vi "Construct.vi"(7 "ColumnMapping":string[][](array[string]), 8 "Error in (no error)":errorcluster, 9 "Table":string, 10 "Database":T1) -> (0 "Error out":errorcluster, 3 "LogWriterDb out":refnum<class "LogWriterDb.lvclass">)   [LabVIEW 2011, in "LogWriterDb.lvclass"]
uses:
  LogWriterDb.lvclass
  <vilib>/addons/database/Connection.llb/Conn ObjectReference.ctl
  LogWriterDb.lvclass/LogWriterDb.ctl
  <vilib>/addons/database/NI_Database_API.lvlib
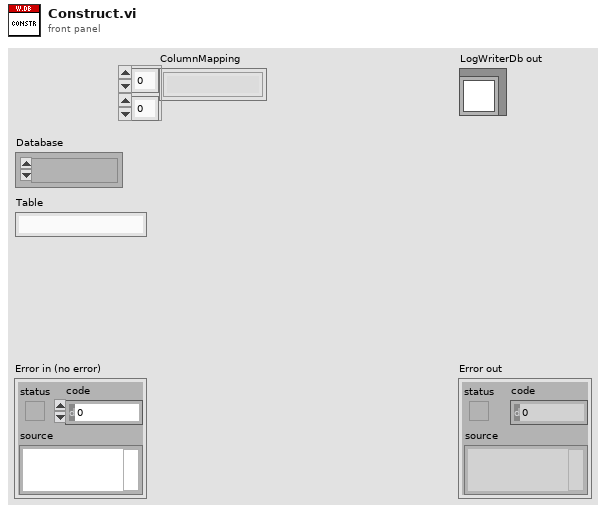
[diagram p1: front panel]
types:
  T1 = typedef "NI_Database_API.lvlib/Conn ObjectReference.ctl" = refnum<k1>
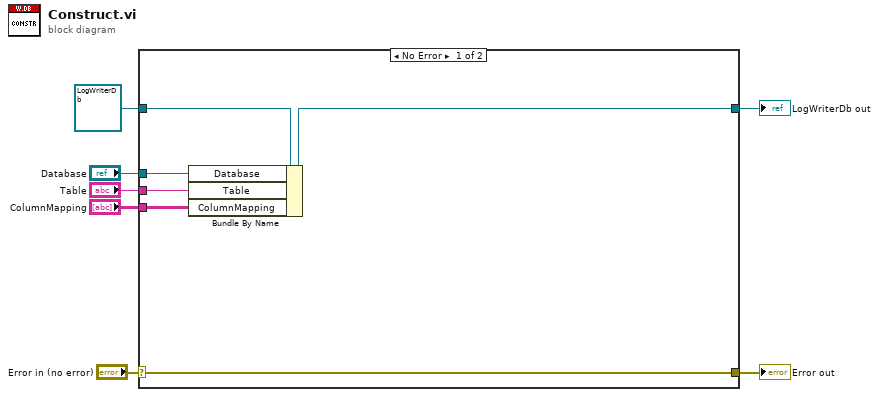
[diagram p0: block diagram]
diagram:
  n1 = case shown="No Error" "Error in (no error)" {
    selector: "Error in (no error)" -> [w13 w15]
    tunnel: [w13 w15] -> w6
    tunnel: [w10 w14] -> w5
    tunnel: refnum<class "LogWriterDb.lvclass"> refnum ("LogWriterDb in") -> [w11 w14]
    tunnel: "Database" -> [w12 _]
    tunnel: "Table" -> [w9 _]
    tunnel: "ColumnMapping" -> [w8 _]
    frame No Error {
      n2 = Bundle By Name(cluster=w11, "Database"=w12, "Table"=w9, "ColumnMapping"=w8) -> (w10:refnum<class "LogWriterDb.lvclass">)
    }
    frame Error {
    }
  }
  "Error out" <- w6
  "LogWriterDb out" <- w5
